vi "Main.vi"() -> ()   [LabVIEW 2021]
uses:
  Controls/App Data.ctl
  Controls/UI References.ctl
  Controls/Channel Selection/Volt Chl.ctl
  <vilib>/Analysis/baseanly.llb/Mean (DBL).vi
  <vilib>/DAQmx/read.llb/DAQmx Read (Analog 1D Wfm NChan NSamp).vi
  <vilib>/DAQmx/write.llb/DAQmx Write (Analog DBL 1Chan 1Samp).vi
  <extravilib>/ChannelInstances/Stream-a[.](wfm(dbl))/Read With Abort.vi
  <extravilib>/ChannelInstances/Stream-a[.](wfm(dbl))/Write With Abort.vi
  <extravilib>/ChannelInstances/Stream-a[.](wfm(dbl))/EndpointRead.vi
  <extravilib>/ChannelInstances/Stream-a[.](wfm(dbl))/Endpoint.vi
  <extravilib>/ChannelInstances/Stream-a[.](wfm(dbl))/Instantiate.vi
  <extravilib>/ChannelInstances/Event Messenger-c(str,var,var)/Instantiate.vi
  <extravilib>/ChannelInstances/Event Messenger-c(str,var,var)/))Channel.vi
  <extravilib>/ChannelInstances/Stream-a[.](wfm(dbl))/)Channel.vi
  <resource>/ChannelSupport/_ChannelSupport/WaitIfNeeded.vi
  <vilib>/DAQmx/miscellaneous.llb/DAQmx Fill In Error Info.vi
  <vilib>/DAQmx/create/channels.llb/DAQmx Create Channel (AO-Voltage-Basic).vi
  <vilib>/DAQmx/create/channels.llb/DAQmx Create Channel (AI-Voltage-Basic).vi
  <vilib>/DAQmx/configure/timing.llb/DAQmx Timing (Sample Clock).vi
  <extravilib>/ChannelInstances/Stream-a[.](wfm(dbl)).lvlib
  <resource>/objmgr/daqmx.rc
  <vilib>/Analysis/NI_AALBase.lvlib
  <extravilib>/ChannelInstances/Event Messenger-c(str,var,var).lvlib
panel:
  out "Boolean":bool=TRUE
  out "x >= y? 2":bool
  out "x >= y?":bool
  out "Calibration State":enum16{"Idle", "Delay", "Voltage", "Response"}(ring)
  in  "Response (ms)":dbl
  in  "Voltage Time (ms)":dbl
  in  "Delay (ms)":dbl
  out "File Path":path
  out "Bridge OP":dbl
  out "Shunt Voltage":dbl
  out "Recording?":bool
  in  "Supplied Voltage":dbl(slide) scale=0.0..5.0
  out "Current Supplied Voltage":dbl
  out "Waveform Graph":waveform(dbl)[](graph)
  in  "Start":bool
  in  "Device Name":tag
  in  "Sample Rate S/s":i32=100
  in  "Select AO Channel":enum16{"0", "1"}(ring)
  in  "Select Channels":bool
  in  "Stop":bool
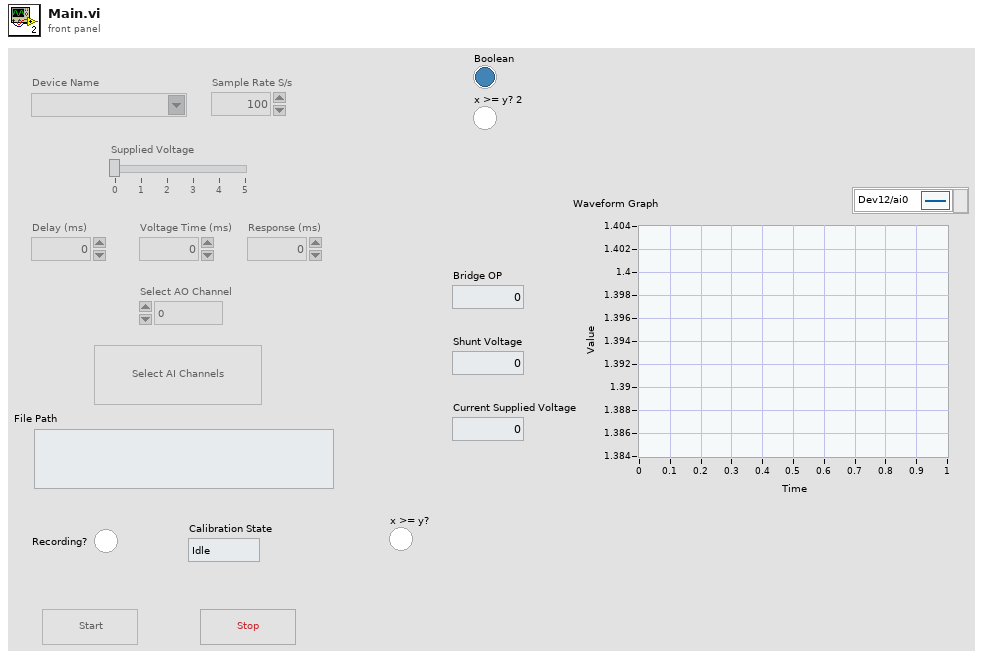
[diagram p1: front panel]
types:
  T1 = typedef "UI References.ctl" = cluster{"Device Name":refnum<vi>, "Sample Rate S/s":refnum<vi>, "Supplied Voltage":refnum<vi>, "Delay (ms)":refnum<vi>, "Voltage Time (ms)":refnum<vi>, "Response (ms)":refnum<vi>, "Select AO Channel":refnum<vi>, "Select Channels":refnum<vi>, "File Path":refnum<vi>, "Recording?":refnum<vi>, "Calibration State":refnum<vi>, "Start":refnum<vi>, "Stop":refnum<vi>, "Bridge OP":refnum<vi>, "Shunt Voltage":refnum<vi>, "Current Supplied Voltage ":refnum<vi>, "Waveform Graph":refnum<vi>}
  T2 = typedef "App Data.ctl" = cluster{"File Refnum":refnum<file>, "AI task":refnum<k21>, "AO task":refnum<k21>, "Sample rate":i32, "Delay (ms)":u32, "Voltage Time (ms)":u32, "Response (ms)":u32, "Supplied Voltage (V)":dbl, "Phase Start Tick (ms)":u32, "Calibration State":enum16{"Idle", "Delay", "Voltage", "Response"}}
  T3 = typedef "Event Messenger-c(str,var,var).lvlib/))Channel.ctl" = refnum<queue>
  T4 = typedef "Volt Chl.ctl" = cluster{"Index":i32[], "Chl Name":string[], "Scale":dbl[], "Offset":dbl[], "Sample Rate":i32, "Device Name":tag, "Channel":tag, "AO Channel":tag}
  T5 = typedef "Stream-a[.](wfm(dbl)).lvlib/)Channel.ctl" = refnum<queue>
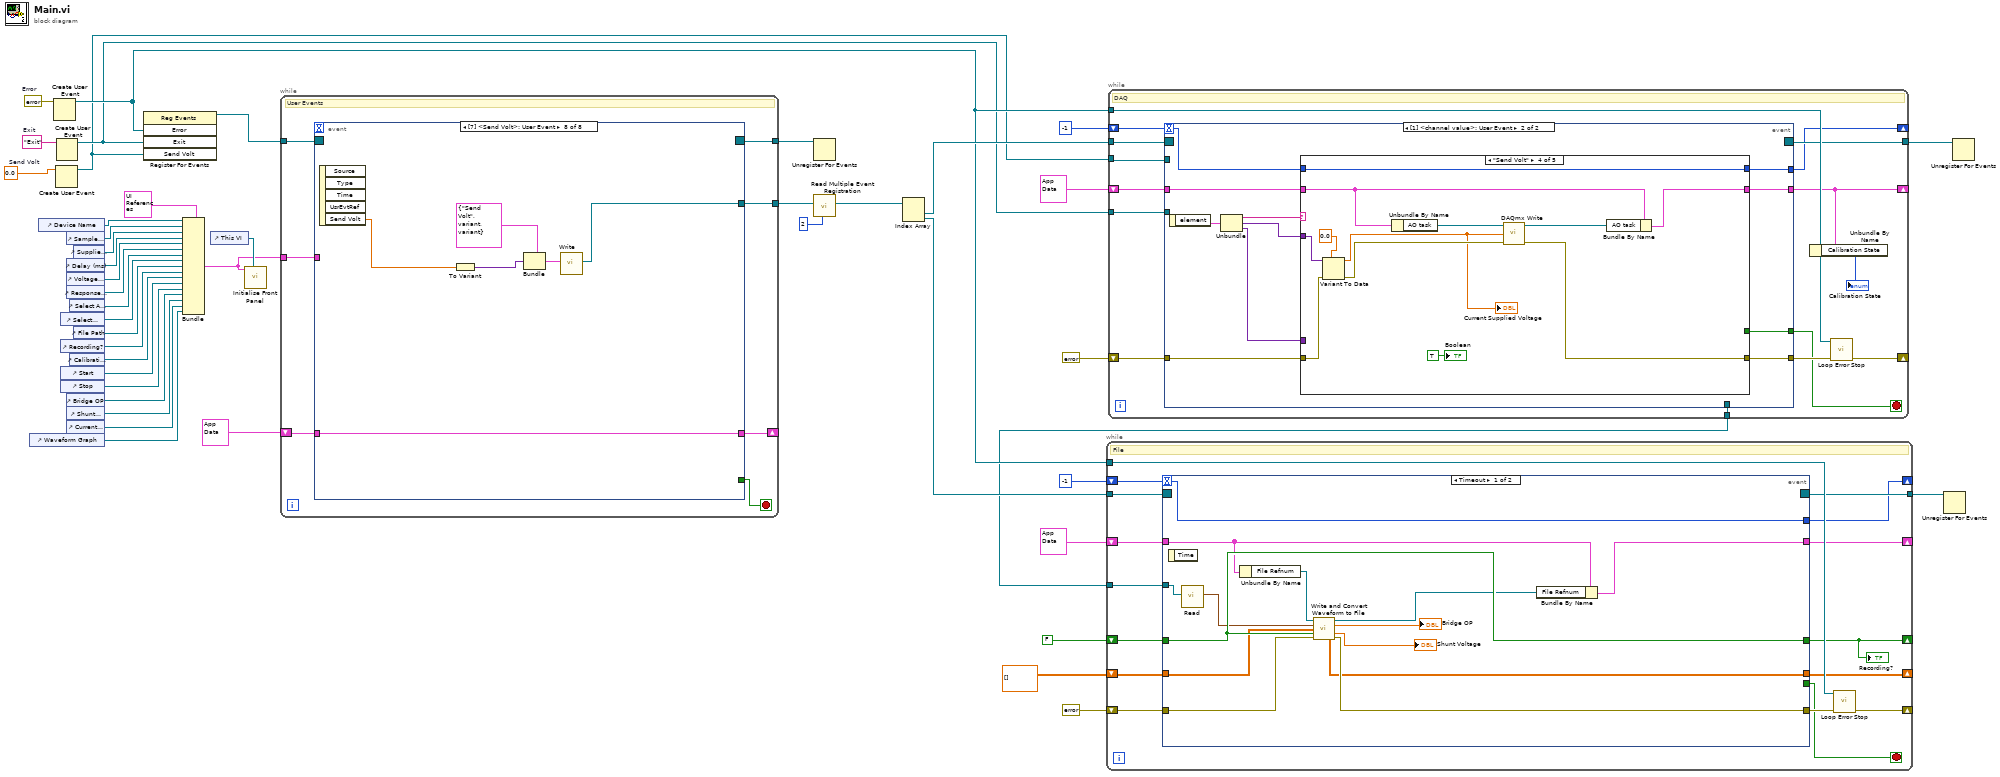
[diagram p0: block diagram]
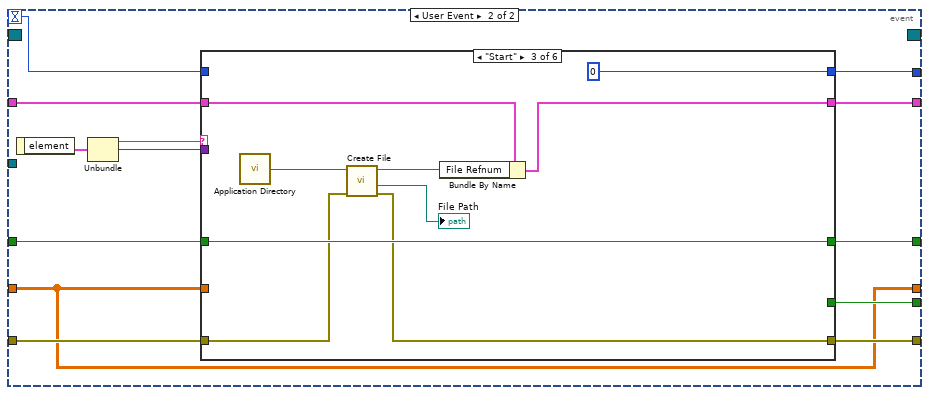
[diagram p2: hidden frame]
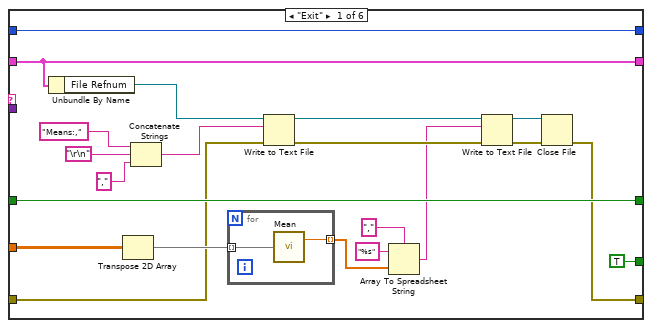
[diagram p3: hidden frame]
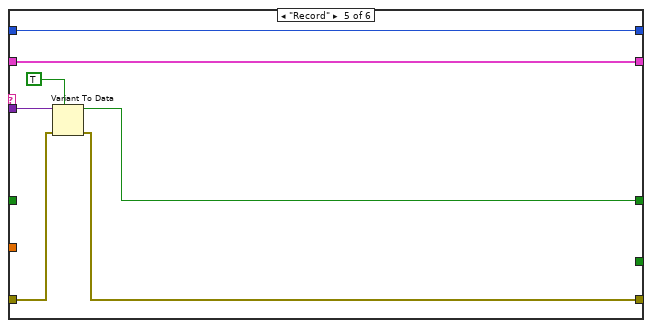
[diagram p6: hidden frame]
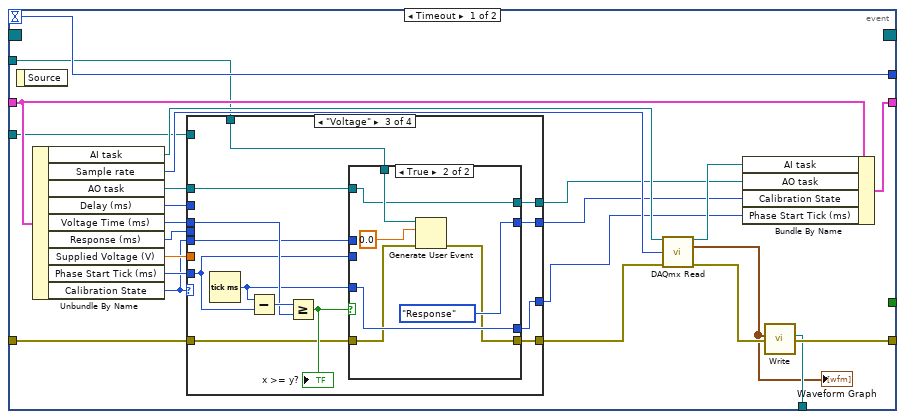
[diagram p8: hidden frame]
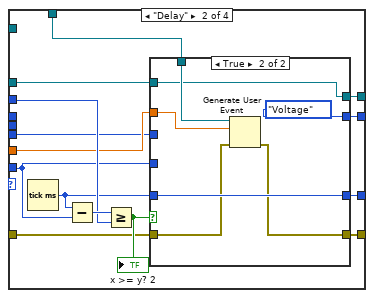
[diagram p10: hidden frame]
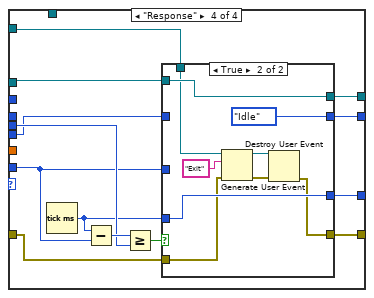
[diagram p13: hidden frame]
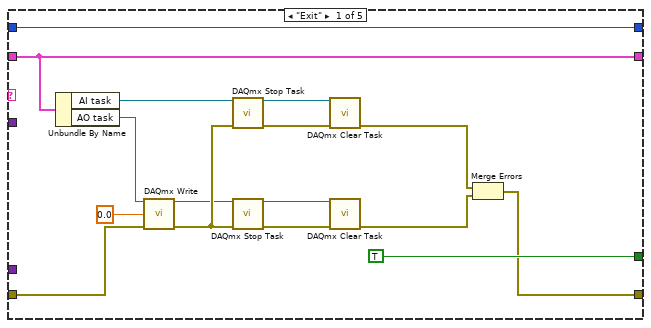
[diagram p15: hidden frame]
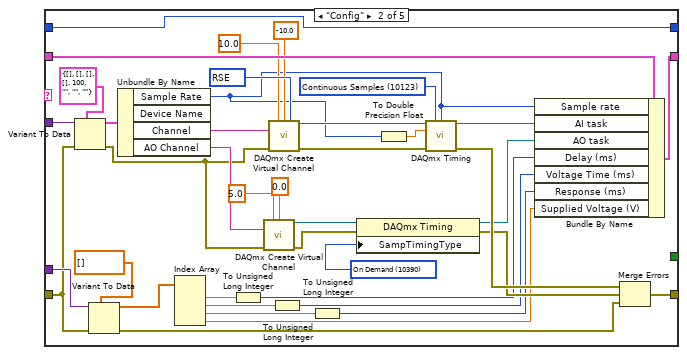
[diagram p16: hidden frame]
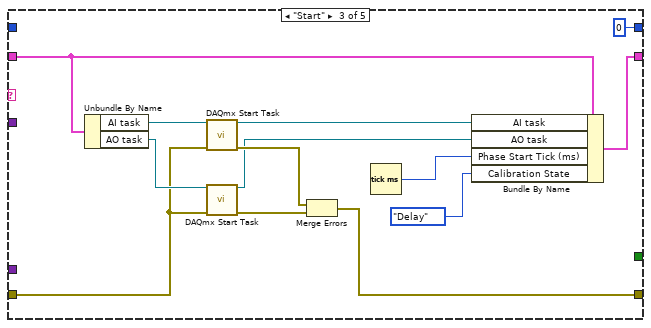
[diagram p17: hidden frame]
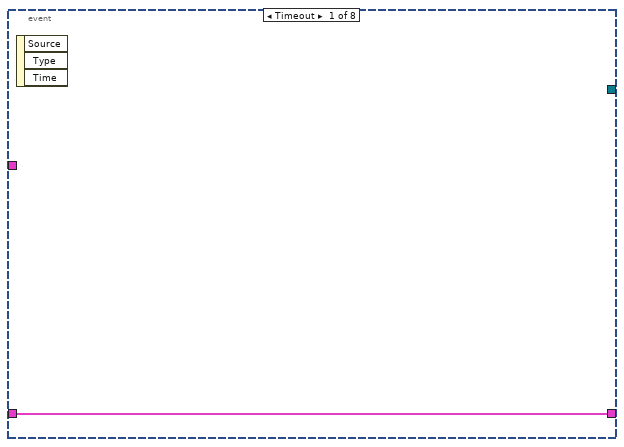
[diagram p19: hidden frame]
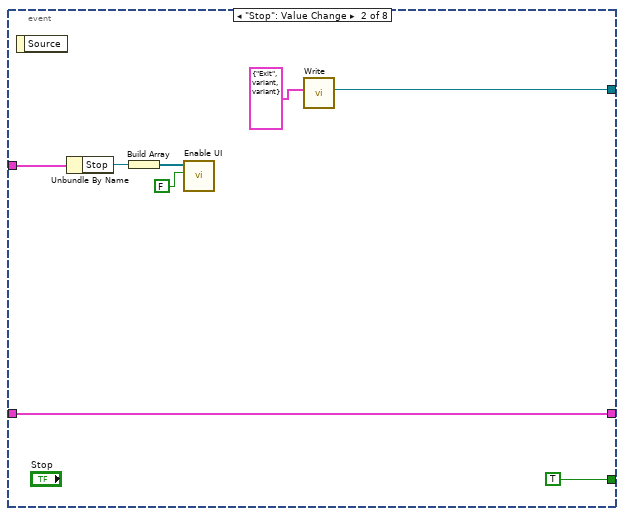
[diagram p20: hidden frame]
diagram:
  w2 = 0.0  # Send Volt
  w4 = "Exit"  # Exit
  w43 = errorcluster {"status"=FALSE, "code"=0, "source"=""}  # Error
  n1 = control-ref of="Waveform Graph"() -> (w6:refnum<vi>)
  n2 = control-ref of="Device Name"() -> (w22:refnum<vi>)
  n3 = Create User Event(user event datatype=w43) -> (user event=w33:refnum<user-event>)  [unwired: 1 in, 1 out]
  n4 = Create User Event(user event datatype=w2) -> (user event=w1:refnum<user-event>)  [unwired: 1 in, 1 out]
  n5 = Create User Event(user event datatype=w4) -> (user event=w3:refnum<user-event>)  [unwired: 1 in, 1 out]
  n6 = control-ref of="Select Channels"() -> (w15:refnum<vi>)
  n7 = control-ref of="Recording?"() -> (w13:refnum<vi>)
  n8 = control-ref of="Start"() -> (w11:refnum<vi>)
  n9 = control-ref of="Stop"() -> (w10:refnum<vi>)
  n10 = control-ref of="Sample Rate S/s"() -> (w21:refnum<vi>)
  n11 = control-ref of="Delay (ms)"() -> (w19:refnum<vi>)
  n12 = control-ref of="Voltage Time (ms)"() -> (w18:refnum<vi>)
  n13 = control-ref of="Response (ms)"() -> (w17:refnum<vi>)
  n14 = control-ref of="Bridge OP"() -> (w9:refnum<vi>)
  n15 = control-ref of="Shunt Voltage"() -> (w8:refnum<vi>)
  n16 = control-ref of="Current Supplied Voltage"() -> (w7:refnum<vi>)
  n17 = control-ref of="Select AO Channel"() -> (w16:refnum<vi>)
  n18 = control-ref of="Calibration State"() -> (w12:refnum<vi>)
  n19 = control-ref of="Supplied Voltage"() -> (w20:refnum<vi>)
  n20 = control-ref of="File Path"() -> (w14:refnum<vi>)
  n21 = register-events(w33, w3, w1) -> (reference out=w42:refnum<event-registration>)  [unwired: 2 in, 1 out]
  n22 = Bundle(cluster=T1 {"Device Name"=refnum, "Sample Rate S/s"=refnum, "Supplied Voltage"=refnum, "Delay (ms)"=refnum, "Voltage Time (ms)"=refnum, "Response (ms)"=refnum, "Select AO Channel"=refnum, "Select Channels"=refnum, "File Path"=refnum, "Recording?"=refnum, "Calibration State"=refnum, "Start"=refnum, "Stop"=refnum, "Bridge OP"=refnum, "Shunt Voltage"=refnum, "Current Supplied Voltage "=refnum, "Waveform Graph"=refnum} ("UI Ref"), "Device Name"=w22, "Sample Rate S/s"=w21, "Supplied Voltage"=w20, "Delay (ms)"=w19, "Voltage Time (ms)"=w18, "Response (ms)"=w17, "Select AO Channel"=w16, "Select Channels"=w15, "File Path"=w14, "Recording?"=w13, "Calibration State"=w12, "Start"=w11, "Stop"=w10, "Bridge OP"=w9, "Shunt Voltage"=w8, "Current Supplied Voltage"=w7, "Waveform Graph"=w6) -> (w40:T1)
  n23 = control-ref of="This VI"() -> (w45:refnum<vi>)
  n24 = call "Initialise Front Panel.vi"("This VI"=w45, "UI Ref"=w40) -> ()  [unwired: 9 in, 1 out]
  n25 = while {
    shift-right: [w50] -> _
    shift-left: T2 {"File Refnum"=refnum, "AI task"="", "AO task"="", "Sample rate"=-1, "Delay (ms)"=0, "Voltage Time (ms)"=0, "Response (ms)"=0, "Supplied Voltage (V)"=0.0, "Phase Start Tick (ms)"=0, "Calibration State"=enum."Idle"} ("App Data") -> [w49]
    tunnel: w42 -> [w52]
    tunnel: [w48] -> w41
    tunnel: w40 -> [w47]
    tunnel: [w46] -> w39
    stop <- w51 stop-if-true
    # "User Events"
    n26 = event shown="[7] <Send Volt>: User Event" {
      selector: w52 -> [_ _ _ _ _ _ _ _]
      dyn-events: [_ _ _ _ _ _ _ _] -> w48
      timeout: _ -> [_ _ _ _ _ _ _ _]
      tunnel: [_ TRUE TRUE TRUE TRUE _ _ _] -> w51
      tunnel: [w53 w60 w64 w67 w72 w75 w117 w119] -> w50
      tunnel: w49 -> [w53 w60 w64 w67 w72 w75 w117 w119]
      tunnel: w47 -> [_ w59 _ _ _ w94 w118 _]
      tunnel: [_ w54 w62 w68 w70 w95 w113 w120] -> w46
      event Timeout {
        n27 = event-data() -> ()  [unwired: 1 in, 3 out]
      }
      event "Stop": Value Change {
        n28 = event-data() -> ()  [unwired: 1 in, 1 out]
        n29 = Unbundle By Name(w59) -> ("Stop"=w58:refnum<vi>)
        n30 = Build Array(w58) -> (w57:refnum<vi>[])
        n31 = call "Enable UI.vi"("Enable?"=FALSE, "output cluster"=w57) -> ()  [unwired: 9 in, 1 out]
        n32 = call <extravilib>:"Write.vi"("element"=cluster{string, variant, variant} {"Exit", variant, variant}) -> ("channel"=w54:T3)  [unwired: 9 in, 1 out]
      }
      event User Event {
        n33 = event-data() -> ()  [unwired: 1 in, 1 out]
        n34 = call <extravilib>:"Write.vi"("element"=cluster{string, variant, variant} {"Exit", variant, variant}) -> ("channel"=w62:T3)  [unwired: 9 in, 1 out]
      }
      event User Event {
        n35 = event-data() -> ()  [unwired: 1 in, 4 out]
        n36 = call <extravilib>:"Write.vi"("element"=cluster{string, variant, variant} {"Exit", variant, variant}) -> ("channel"=w68:T3)  [unwired: 9 in, 1 out]
      }
      event Panel Close? {
        n37 = event-data() -> ()  [unwired: 1 in, 4 out]
        n38 = call <extravilib>:"Write.vi"("element"=cluster{string, variant, variant} {"Exit", variant, variant}) -> ("channel"=w70:T3)  [unwired: 9 in, 1 out]
        n39 = event-data() -> ()  [unwired: 2 in, 1 out]
      }
      event "Select Channels": Value Change {
        n40 = event-data() -> ()  [unwired: 1 in, 6 out]
        n41 = Unbundle By Name(w94) -> ("Device Name"=w89:refnum<vi>, "Sample Rate S/s"=w88:refnum<vi>, "Supplied Voltage"=w87:refnum<vi>, "Delay (ms)"=w86:refnum<vi>, "Voltage Time (ms)"=w85:refnum<vi>, "Response (ms)"=w84:refnum<vi>, "Select AO Channel"=w83:refnum<vi>, "Select Channels"=w82:refnum<vi>, "Start"=w81:refnum<vi>)
        n42 = call "DAQ Channel Dlg_V0.vi"("DAQ Sample Rate (S/s)"="Sample Rate S/s", "AO Channel"="Select AO Channel", "Device Name"="Device Name") -> ("Chl Infor"=w97:variant)  [unwired: 8 in]
        n43 = Build Array(w81) -> (w91:refnum<vi>[])
        n44 = Build Array(w89, w88, w87, w86, w85, w84, w83, w82) -> (w93:refnum<vi>[])
        n45 = Build Array("Delay (ms)", "Voltage Time (ms)", "Response (ms)", "Supplied Voltage") -> (w77:dbl[])
        n46 = To Variant(anything=w77) -> (Variant=w76:variant)
        n47 = Bundle(cluster=cluster{string, variant, variant} {"Config", variant, variant}, w97, w76) -> (w96:cluster{string, variant, variant})  [unwired: 1 in]
        n48 = call <extravilib>:"Write.vi"("element"=w96) -> ("channel"=w95:T3)  [unwired: 9 in, 1 out]
        n49 = call "Enable UI.vi"("Enable?"=FALSE, "output cluster"=w93) -> ()  [unwired: 9 in, 1 out]
        n50 = call "Enable UI.vi"("Enable?"=TRUE, "output cluster"=w91) -> ()  [unwired: 9 in, 1 out]
      }
      event "Start": Value Change {
        n51 = event-data() -> ()  [unwired: 1 in, 1 out]
        n52 = Unbundle By Name(w118) -> ("File Path"=w110:refnum<vi>, "Recording?"=w109:refnum<vi>, "Calibration State"=w108:refnum<vi>, "Stop"=w107:refnum<vi>, "Bridge OP"=w106:refnum<vi>, "Shunt Voltage"=w105:refnum<vi>, "Current Supplied Voltage"=w104:refnum<vi>, "Waveform Graph"=w103:refnum<vi>, "Start"=w102:refnum<vi>)
        n53 = Build Array(w102) -> (w111:refnum<vi>[])
        n54 = Build Array(w110, w109, w108, w107, w106, w105, w104, w103) -> (w112:refnum<vi>[])
        n55 = call <extravilib>:"Write.vi"("element"=cluster{string, variant, variant} {"Start", variant, variant}) -> ("channel"=w113:T3)  [unwired: 9 in, 1 out]
        n56 = call "Enable UI.vi"("Enable?"=TRUE, "output cluster"=w112) -> ()  [unwired: 9 in, 1 out]
        n57 = call "Enable UI.vi"("Enable?"=FALSE, "output cluster"=w111) -> ()  [unwired: 9 in, 1 out]
      }
      event User Event {
        n58 = event-data() -> ("Send Volt"=w123:dbl)  [unwired: 1 in, 4 out]
        n59 = To Variant(anything=w123) -> (Variant=w122:variant)
        n60 = Bundle(cluster=cluster{string, variant, variant} {"Send Volt", variant, variant}, w122) -> (w121:cluster{string, variant, variant})  [unwired: 2 in]
        n61 = call <extravilib>:"Write.vi"("element"=w121) -> ("channel"=w120:T3)  [unwired: 9 in, 1 out]
      }
    }
  }
  n62 = Unregister For Events(event registration refnum=w41) -> ()  [unwired: 1 in, 1 out]
  n63 = call <extravilib>:"Read Multiple Event Registration.vi"("number of event structures"=u16 2, "channel"=w39) -> ("event registration refnums"=w37:refnum<event-registration>[])  [unwired: 9 in]
  n64 = Index Array(array=w37) -> (element #1=w36:refnum<event-registration>, element #2=w31:refnum<event-registration>)  [unwired: 2 in]
  n65 = while {
    tunnel: w36 -> [w139]
    shift-right: [w127] -> _
    shift-left: T2 {"File Refnum"=refnum, "AI task"="", "AO task"="", "Sample rate"=-1, "Delay (ms)"=0, "Voltage Time (ms)"=0, "Response (ms)"=0, "Supplied Voltage (V)"=0.0, "Phase Start Tick (ms)"=0, "Calibration State"=enum."Idle"} ("App Data") -> [w138]
    shift-right: [w137] -> _
    shift-left: errorcluster {"status"=FALSE, "code"=0, "source"=""} ("error in (no error)") -> [w136]
    tunnel: w33 -> [w134]
    tunnel: [w132] -> w29
    shift-right: [w130] -> _
    shift-left: -1 -> [w131]
    tunnel: [w129] -> w25
    tunnel: w3 -> [w128]
    tunnel: w1 -> [w125]
    stop <- w133 stop-if-true
    # "DAQ"
    n66 = event shown="[1] <channel value>: User Event" {
      selector: w139 -> [_ _]
      dyn-events: [_ _] -> w132
      timeout: w131 -> [w162 w244]
      tunnel: w138 -> [w150 w247]
      tunnel: w136 -> [w154 w250]
      tunnel: [w161 w249] -> w135
      tunnel: [w149 w248] -> w127
      tunnel: [_ w246] -> w133
      tunnel: [w162 w243] -> w130
      tunnel: [w159 _] -> w129
      tunnel: w128 -> [w141 _]
      tunnel: w125 -> [w140 _]
      event Timeout {
        n67 = event-data() -> ()  [unwired: 1 in, 1 out]
        n68 = Unbundle By Name(w150) -> ("AI task"=w158:refnum<k21>, "Sample rate"=w157:i32, "AO task"=w153:refnum<k21>, "Delay (ms)"=w155:u32, "Voltage Time (ms)"=w144:u32, "Response (ms)"=w142:u32, "Supplied Voltage (V)"=w152:dbl, "Phase Start Tick (ms)"=w156:u32, "Calibration State"=w145:enum16{"Idle", "Delay", "Voltage", "Response"})
        n69 = case shown="\"Voltage\"" w145 {
          tunnel: w156 -> [w164 w169 w193 w217]
          tunnel: w155 -> [_ w178 _ _]
          tunnel: w154 -> [w163 w177 w199 w222]
          tunnel: w153 -> [w166 w176 w201 w223]
          tunnel: w152 -> [_ w175 _ _]
          tunnel: [w166 w174 w200 w224] -> w148
          tunnel: [w165 w173 w198 w225] -> w147
          tunnel: [w164 w172 w196 w219] -> w146
          tunnel: w145 -> [w165 w170 w194 w218]
          tunnel: w144 -> [_ _ w203 _]
          tunnel: [w163 w168 w195 w221] -> w143
          tunnel: w142 -> [_ _ _ w227]
          tunnel: w141 -> [_ _ _ w216]
          tunnel: w140 -> [_ w167 w192 _]
          frame "Idle", Default {
          }
          frame "Delay" {
            n70 = Tick Count (ms)() -> (millisecond timer value=w171:u32)
            n71 = Subtract(x=w171, y=w169) -> (x-y=w180:u32)
            n72 = Greater Or Equal?(x=w180, y=w178) -> (x >= y?=w179:bool)
            "x >= y? 2" <- w179
            n73 = case shown="True" w179 {
              tunnel: w177 -> [w181 w188]
              tunnel: w176 -> [w184 w185]
              tunnel: w175 -> [_ w186]
              tunnel: [w184 w185] -> w174
              tunnel: [w183 enum16{"Idle", "Delay", "Voltage", "Response"}."Voltage" ("Calibration State")] -> w173
              tunnel: [w182 w190] -> w172
              tunnel: w171 -> [_ w190]
              tunnel: w170 -> [w183 _]
              tunnel: w169 -> [w182 _]
              tunnel: [w181 w187] -> w168
              tunnel: w167 -> [_ w189]
              frame False {
              }
              frame True {
                n74 = Generate User Event(user event=w189, event data cluster=w186, error in=w188) -> (error out=w187:errorcluster)  [unwired: 1 in, 1 out]
              }
            }
          }
          frame "Voltage" {
            n75 = Tick Count (ms)() -> (millisecond timer value=w197:u32)
            n76 = Subtract(x=w197, y=w193) -> (x-y=w204:u32)
            n77 = Greater Or Equal?(x=w204, y=w203) -> (x >= y?=w202:bool)
            "x >= y?" <- w202
            n78 = case shown="True" w202 {
              tunnel: w201 -> [w208 w209]
              tunnel: [w208 w209] -> w200
              tunnel: w199 -> [w205 w211]
              tunnel: [w207 enum16{"Idle", "Delay", "Voltage", "Response"}."Response" ("Calibration State")] -> w198
              tunnel: w197 -> [_ w214]
              tunnel: [w206 w214] -> w196
              tunnel: [w205 w210] -> w195
              tunnel: w194 -> [w207 _]
              tunnel: w193 -> [w206 _]
              tunnel: w192 -> [_ w213]
              frame False {
              }
              frame True {
                n79 = Generate User Event(user event=w213, event data cluster=0.0 ("data"), error in=w211) -> (error out=w210:errorcluster)  [unwired: 1 in, 1 out]
              }
            }
          }
          frame "Response" {
            n80 = Tick Count (ms)() -> (millisecond timer value=w220:u32)
            n81 = Subtract(x=w220, y=w217) -> (x-y=w228:u32)
            n82 = Greater Or Equal?(x=w228, y=w227) -> (x >= y?=w226:bool)
            n83 = case shown="True" w226 {
              tunnel: [w231 enum16{"Idle", "Delay", "Voltage", "Response"}."Idle" ("Calibration State")] -> w225
              tunnel: [w232 w240] -> w224
              tunnel: w223 -> [w232 w240]
              tunnel: w222 -> [w229 w237]
              tunnel: [w229 w233] -> w221
              tunnel: w220 -> [_ w239]
              tunnel: [w230 w239] -> w219
              tunnel: w218 -> [w231 _]
              tunnel: w217 -> [w230 _]
              tunnel: w216 -> [_ w238]
              frame False {
              }
              frame True {
                n84 = Generate User Event(user event=w238, event data cluster="Exit" ("event data"), error in=w237) -> (user event out=w234:refnum<user-event>, error out=w235:errorcluster)  [unwired: 1 in]
                n85 = Destroy User Event(user event=w234, error in=w235) -> (error out=w233:errorcluster)
              }
            }
          }
        }
        n86 = call-poly <vilib>:"DAQmx Read.vi"("task/channels in"=w158, "number of samples per channel"=w157, "error in"=w143) -> ("task out"=w160:refnum<k21>, "data"=w151:waveform(dbl)[], "error out"=w161:errorcluster)  [unwired: 10 in]
        "Waveform Graph" <- w151
        n87 = Bundle By Name(cluster=w150, "AI task"=w160, "AO task"=w148, "Calibration State"=w147, "Phase Start Tick (ms)"=w146) -> (w149:T2)
        n88 = call <extravilib>:"Write.vi"("element"=w151) -> ("channel"=w159:T5)  [unwired: 8 in, 2 out]
      }
      event User Event {
        n89 = event-data() -> ("element"=w252:cluster{string, variant, variant})  [unwired: 1 in]
        n90 = Unbundle(w252) -> (w251:string, w245:variant, w242:variant)
        n91 = case shown="\"Send Volt\"" w251 {
          tunnel: w250 -> [w256 w279 w318 w324 w334]
          tunnel: [w259 w300 w316 w330 w334] -> w249
          tunnel: [w267 w296 w311 w327 w335] -> w248
          tunnel: w247 -> [w267 w298 w310 w329 w335]
          tunnel: [TRUE _ _ _ _] -> w246
          tunnel: w245 -> [_ w307 _ w326 _]
          tunnel: w244 -> [w258 w282 _ w332 w333]
          tunnel: [w258 w282 0 w332 w333] -> w243
          tunnel: w242 -> [_ w280 _ _ _]
          frame "Exit" {
            n92 = Unbundle By Name(w267) -> ("AI task"=w266:refnum<k21>, "AO task"=w257:refnum<k21>)
            n93 = call-poly <vilib>:"DAQmx Write.vi"("task/channels in"=w257, "data"=0.0, "error in"=w256) -> ("task out"=w254:refnum<k21>, "error out"=w255:errorcluster)  [unwired: 10 in, 1 out]
            n94 = call <vilib>:"DAQmx Stop Task.vi"("task/channels in"=w266, "error in"=w255) -> ("task out"=w265:refnum<k21>, "error out"=w262:errorcluster)  [unwired: 12 in]
            n95 = call <vilib>:"DAQmx Stop Task.vi"("task/channels in"=w254, "error in"=w255) -> ("task out"=w264:refnum<k21>, "error out"=w263:errorcluster)  [unwired: 12 in]
            n96 = call <vilib>:"DAQmx Clear Task.vi"("task in"=w265, "error in"=w262) -> ("error out"=w261:errorcluster)  [unwired: 13 in]
            n97 = call <vilib>:"DAQmx Clear Task.vi"("task in"=w264, "error in"=w263) -> ("error out"=w260:errorcluster)  [unwired: 13 in]
            n98 = Merge Errors(w261, w260) -> (w259:errorcluster)
          }
          frame "Config" {
            w285 = 10390 items=["Sample Clock"=10388, "Burst Handshake"=12548, "Handshake"=10389, "Implicit"=10451, "On Demand"=10390, "Change Detection"=12504, "Pipelined Sample Clock"=14668] ("SampTimingType")
            w292 = 10083 items=["Default"=-1, "RSE"=10083, "NRSE"=10078, "Differential"=10106, "Pseudodifferential"=12529] ("input terminal configuration")
            w293 = 10123 items=["Finite Samples"=10178, "Continuous Samples"=10123, "Hardware Timed Single Point"=12522] ("sample mode")
            n99 = Variant To Data(error in=w279, type=T4 {"Index"=[], "Chl Name"=[], "Scale"=[], "Offset"=[], "Sample Rate"=100, "Device Name"="", "Channel"="", "AO Channel"=""} ("Volt Channel"), Variant=w307) -> (data=w305:T4, error out=w301:errorcluster)
            n100 = Variant To Data(error in=w279, type=dbl[] [], Variant=w280) -> (data=w276:dbl[], error out=w278:errorcluster)
            n101 = Unbundle By Name(w305) -> ("Sample Rate"=w281:i32, "Channel"=w304:tag, "AO Channel"=w303:tag)  [unwired: 1 out]
            n102 = Index Array(array=w276) -> (element #1=w275:dbl, element #2=w274:dbl, element #3=w273:dbl, element #4=w272:dbl)  [unwired: 4 in]
            n103 = To Unsigned Long Integer(number=w275) -> (unsigned 32bit integer=w271:u32)
            n104 = call-poly <vilib>:"DAQmx Create Virtual Channel.vi"("maximum value"=5.0, "minimum value"=0.0, "physical channels"=w303, "error in"=w301) -> ("task out"=w295:refnum<k21>, "error out"=w284:errorcluster)  [unwired: 10 in]
            n105 = call-poly <vilib>:"DAQmx Create Virtual Channel.vi"("maximum value"=10.0, "minimum value"=-10.0, "input terminal configuration"=w292, "physical channels"=w304, "error in"=w301) -> ("task out"=w299:refnum<k21>, "error out"=w302:errorcluster)  [unwired: 9 in]
            n106 = To Unsigned Long Integer(number=w274) -> (unsigned 32bit integer=w270:u32)
            n107 = To Unsigned Long Integer(number=w273) -> (unsigned 32bit integer=w269:u32)
            n108 = property class="DAQmx Timing"(reference=w295, error in=w284, "SampTimingType"=w285) -> (reference out=w286:refnum<k21>, error out=w283:errorcluster)
            n109 = To Double Precision Float(number=w281) -> (double precision float=w289:dbl)
            n110 = call-poly <vilib>:"DAQmx Timing.vi"("task/channels in"=w299, "sample mode"=w293, "samples per channel"=w281, "rate"=w289, "error in"=w302) -> ("task out"=w297:refnum<k21>, "error out"=w294:errorcluster)  [unwired: 9 in]
            n111 = Bundle By Name(cluster=w298, "Sample rate"=w281, "AI task"=w297, "AO task"=w286, "Delay (ms)"=w271, "Voltage Time (ms)"=w270, "Response (ms)"=w269, "Supplied Voltage (V)"=w272) -> (w296:T2)
            n112 = Merge Errors(w294, w283, w278) -> (w300:errorcluster)
          }
          frame "Start" {
            n113 = Unbundle By Name(w310) -> ("AI task"=w320:refnum<k21>, "AO task"=w319:refnum<k21>)
            n114 = call <vilib>:"DAQmx Start Task.vi"("task/channels in"=w320, "error in"=w318) -> ("task out"=w315:refnum<k21>, "error out"=w317:errorcluster)  [unwired: 12 in]
            n115 = call <vilib>:"DAQmx Start Task.vi"("task/channels in"=w319, "error in"=w318) -> ("task out"=w314:refnum<k21>, "error out"=w313:errorcluster)  [unwired: 12 in]
            n116 = Merge Errors(w317, w313) -> (w316:errorcluster)
            n117 = Tick Count (ms)() -> (millisecond timer value=w309:u32)
            n118 = Bundle By Name(cluster=w310, "AI task"=w315, "AO task"=w314, "Phase Start Tick (ms)"=w309, "Calibration State"=enum16{"Idle", "Delay", "Voltage", "Response"}."Delay") -> (w311:T2)
          }
          frame "Send Volt" {
            n119 = Variant To Data(error in=w324, type=0.0, Variant=w326) -> (data=w322:dbl, error out=w323:errorcluster)
            "Current Supplied Voltage" <- w322
            n120 = Unbundle By Name(w329) -> ("AO task"=w331:refnum<k21>)
            n121 = call-poly <vilib>:"DAQmx Write.vi"("task/channels in"=w331, "data"=w322, "error in"=w323) -> ("task out"=w328:refnum<k21>, "error out"=w330:errorcluster)  [unwired: 10 in, 1 out]
            n122 = Bundle By Name(cluster=w329, "AO task"=w328) -> (w327:T2)
            "Boolean" <- TRUE
          }
          frame Default {
          }
        }
      }
    }
    n123 = Unbundle By Name(w127) -> ("Calibration State"=→"Calibration State":enum16{"Idle", "Delay", "Voltage", "Response"})
    n124 = call "Loop Error Stop.vi"("error in"=w135, "user event"=w134) -> ("error out"=w137:errorcluster)  [unwired: 9 in]
  }
  n125 = while {
    tunnel: w31 -> [w351]
    shift-right: [w345] -> _
    shift-left: T2 {"File Refnum"=refnum, "AI task"="", "AO task"="", "Sample rate"=-1, "Delay (ms)"=0, "Voltage Time (ms)"=0, "Response (ms)"=0, "Supplied Voltage (V)"=0.0, "Phase Start Tick (ms)"=0, "Calibration State"=enum."Idle"} ("App Data") -> [w350]
    shift-right: [w349] -> _
    shift-left: errorcluster {"status"=FALSE, "code"=0, "source"=""} ("error in (no error)") -> [w348]
    tunnel: w33 -> [w346]
    tunnel: [w343] -> w28
    shift-right: [w341] -> _
    shift-left: -1 -> [w342]
    tunnel: w25 -> [w340]
    shift-right: [w338] -> _
    shift-left: FALSE -> [w339]
    shift-right: [w336] -> _
    shift-left: dbl[][] [] -> [w337]
    stop <- w344 stop-if-true
    # "File"
    n126 = event shown="[0] Timeout" {
      selector: w351 -> [_ _]
      dyn-events: [_ _] -> w343
      timeout: w342 -> [w364 w371]
      tunnel: w350 -> [w356 w373]
      tunnel: w348 -> [w361 w376]
      tunnel: [w362 w375] -> w347
      tunnel: [w354 w374] -> w345
      tunnel: [_ w372] -> w344
      tunnel: [w364 w370] -> w341
      tunnel: w340 -> [w365 _]
      tunnel: w339 -> [w363 w368]
      tunnel: [w363 w369] -> w338
      tunnel: w337 -> [w352 w366]
      tunnel: [w353 w366] -> w336
      event Timeout {
        n127 = event-data() -> ()  [unwired: 1 in, 1 out]
        n128 = call <extravilib>:"Read.vi"("channel"=w365) -> ("element"=w360:waveform(dbl)[])  [unwired: 6 in, 4 out]
        n129 = Unbundle By Name(w356) -> ("File Refnum"=w357:refnum<file>)
        n130 = call "Write and Convert Waveform to File.vi"("File Refnum"=w357, "Waveform"=w360, "Prev Array"=w352, "Record?"=w363, "error in"=w361) -> ("File Refnum Out"=w355:refnum<file>, "Voltage Out"=→"Bridge OP":dbl, "Flow Out"=→"Shunt Voltage":dbl, "Volt & Flow array"=w353:dbl[][], "error out"=w362:errorcluster)  [unwired: 6 in]
        n131 = Bundle By Name(cluster=w356, "File Refnum"=w355) -> (w354:T2)
      }
      event User Event {
        n132 = event-data() -> ("element"=w378:cluster{string, variant, variant})  [unwired: 1 in]
        n133 = Unbundle(w378) -> (w377:string, w367:variant)  [unwired: 1 out]
        n134 = case shown="\"Start\"" w377 {
          tunnel: w376 -> [w386 w404 w412 w417 w422 w428]
          tunnel: [w395 w404 w411 w417 w421 w428] -> w375
          tunnel: [w396 w405 w406 w418 w425 w429] -> w374
          tunnel: w373 -> [w396 w405 w408 w418 w425 w429]
          tunnel: [TRUE _ _ _ _ _] -> w372
          tunnel: w371 -> [w398 w403 _ w416 w424 w427]
          tunnel: [w398 w403 0 w416 w424 w427] -> w370
          tunnel: [w397 w402 w413 w415 w419 w426] -> w369
          tunnel: w368 -> [w397 w402 w413 w415 _ w426]
          tunnel: w367 -> [_ _ _ _ w423 _]
          tunnel: w366 -> [w379 _ _ _ _ _]
          frame "Exit" {
            n135 = Unbundle By Name(w396) -> ("File Refnum"=w387:refnum<file>)
            n136 = Transpose 2D Array(2D array=w379) -> (transposed array=w394:dbl[][])
            n137 = Concatenate Strings "Concatenate Strings"("Means:," ("string"), "\r\n", "," ("string")) -> (w381:string)
            n138 = for {
              tunnel: w394 -> [w401] mode=indexing
              tunnel: [w400] -> w393 mode=indexing
              n139 = call-poly <vilib>:"Mean.vi"("X"=w401) -> ("mean"=w400:dbl)  [unwired: 1 out]
            }
            n140 = Write to Text File(file (use dialog)=w387, text=w381, error in=w386) -> (refnum out=w385:refnum<file>, error out=w384:errorcluster)  [unwired: 1 in, 1 out]
            n141 = Array To Spreadsheet String(delimiter (Tab)=",", array=w393, 3:"%s" ("format string")) -> (spreadsheet string=w380:string)
            n142 = Write to Text File(file (use dialog)=w385, text=w380, error in=w384) -> (refnum out=w383:refnum<file>, error out=w382:errorcluster)  [unwired: 1 in, 1 out]
            n143 = Close File(refnum=w383, error in=w382) -> (error out=w395:errorcluster)  [unwired: 1 out]
          }
          frame "Config" {
          }
          frame "Start" {
            n144 = call <vilib>:"Application Directory.vi"() -> ("Application Directory"=w410:path)
            n145 = call "Create File.vi"("error in"=w412, "Root Path"=w410) -> ("error out"=w411:errorcluster, "File Path Out"=→"File Path":path, "Refnum Out"=w407:refnum<file>)  [unwired: 7 in]
            n146 = Bundle By Name(cluster=w408, "File Refnum"=w407) -> (w406:T2)
          }
          frame "Send Volt" {
          }
          frame "Record" {
            n147 = Variant To Data(error in=w422, type=TRUE, Variant=w423) -> (data=w419:bool, error out=w421:errorcluster)
          }
          frame Default {
          }
        }
      }
    }
    "Recording?" <- w338
    n148 = call "Loop Error Stop.vi"("error in"=w347, "user event"=w346) -> ("error out"=w349:errorcluster)  [unwired: 9 in]
  }
  n149 = Unregister For Events(event registration refnum=w28) -> ()  [unwired: 1 in, 1 out]
  n150 = Unregister For Events(event registration refnum=w29) -> ()  [unwired: 1 in, 1 out]
